vi "UnegisterImagePixelPtr.vi"(8 "error in":errorcluster, 10 "PixelPointer":T1 {"Pixel Pointer" format="%.0x"}, 11 "Image Reference In":T2) -> (0 "error out":errorcluster, 3 "Image Reference Out":T2)   [LabVIEW 2020, in "OpenLvVision_Image.lvlib" / "DataAccess.lvlib"]
doc: "Returns the pixel memory pointer and alignment details."
uses:
  DataAccess.lvlib
  Management/TypeDef/Image.ctl
  TypeDef/PixelPointer.ctl
  Management/Management.lvlib
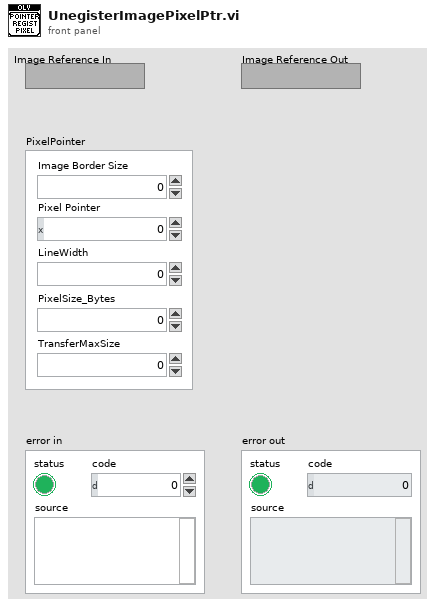
[diagram p1: front panel]
types:
  T1 = typedef "OpenLvVision_Image.lvlib/DataAccess.lvlib/PixelPointer.ctl" = cluster{"Image Border Size":i32, "Pixel Pointer":u64, "LineWidth":i32, "PixelSize_Bytes":i32, "TransferMaxSize":i32}
  T2 = typedef "OpenLvVision_Image.lvlib/Management.lvlib/Image.ctl" = refnum<image>
  T3 = enum32{"Map Pixel Pointer", "Unmap Pixel Pointer", "Get Pixels Infos"}
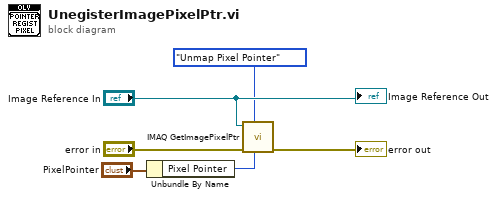
[diagram p0: block diagram]
diagram:
  n1 = Unbundle By Name("PixelPointer") -> ("Pixel Pointer"=w1:u64)
  n2 = call "IMAQ GetImagePixelPtr"("Pixel Pointer in"=w1, "Function"=T3."Unmap Pixel Pointer", "error in (no error)"="error in", "Image"="Image Reference In") -> ("error out"=→"error out":errorcluster)  [unwired: 2 in, 5 out]
  "Image Reference Out" <- "Image Reference In"
